vi "SubVI_SVM_E_calculation.vi"(6 "Y":dbl[][](array[numeric]), 7 "Index":i32, 8 "E":T1, 9 "b":dbl, 10 "K":T1, 11 "Alphas":dbl[][](array[numeric])) -> (0 "alpha[index]":dbl, 1 "y[index]":dbl, 2 "E":T1, 3 "E[index]":dbl)   [LabVIEW 2020]
uses:
  <vilib>/Analysis/Matrix/Datatypes/RealMatrix.ctl
  <vilib>/Analysis/Matrix/Numeric/Conversions/Matrix To Array - RM.vi
  <vilib>/Analysis/Matrix/NI_Matrix.lvlib
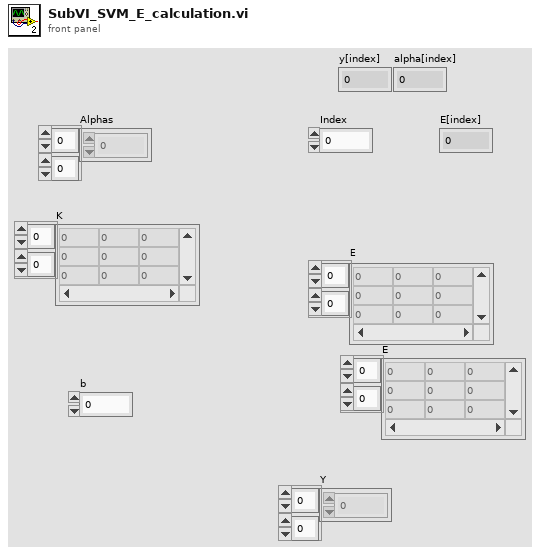
[diagram p1: front panel]
types:
  T1 = typedef "NI_Matrix.lvlib/RealMatrix.ctl" = dbl[][]
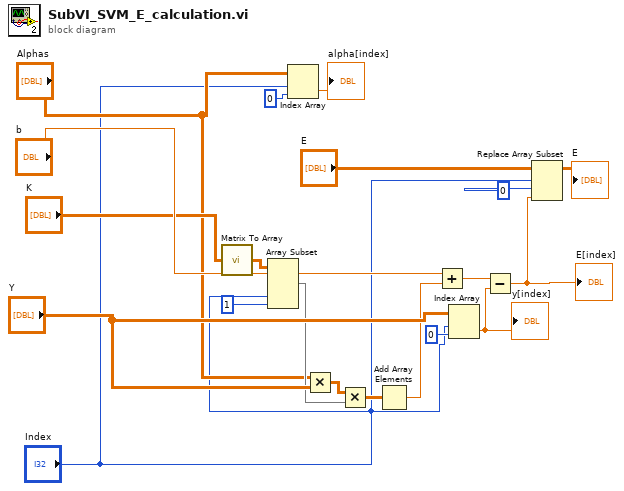
[diagram p0: block diagram]
diagram:
  n1 = call-poly <vilib>:"Matrix To Array.vi"("Real Matrix"="K") -> ("Real 2D Array"=w11:dbl[][])
  n2 = Array Subset(array=w11, index (col)="Index", length (col)=1 ("length")) -> (w13:dbl[][])  [unwired: 2 in]
  n3 = Index Array(array="Alphas", index (row)="Index", index (col)=0 ("disabled index (col)")) -> (element=→"alpha[index]":dbl)
  n4 = Multiply(x="Alphas", y="Y") -> (x*y=w12:dbl[][])
  n5 = Multiply(x=w12, y=w13) -> (x*y=w14:dbl[][])
  n6 = Add Array Elements(numeric array=w14) -> (sum=w16:dbl)
  n7 = Add(x="b", y=w16) -> (x+y=w17:dbl)
  n8 = Index Array(array="Y", index (row)="Index", index (col)=0 ("disabled index (col)")) -> (element=w20:dbl)
  "y[index]" <- w20
  n9 = Subtract(x=w17, y=w20) -> (x-y=w6:dbl)
  "E[index]" <- w6
  n10 = Replace Array Subset(array="E", new element=w6, index (row)="Index", index (col)=0 ("disabled index (col)")) -> (→"E":T1)
